vi "Get XY.vi"(8 "error in":errorcluster, 10 "device name":tag) -> (0 "error out":errorcluster, 2 "Y":dbl, 3 "X":dbl)   [LabVIEW 2015]
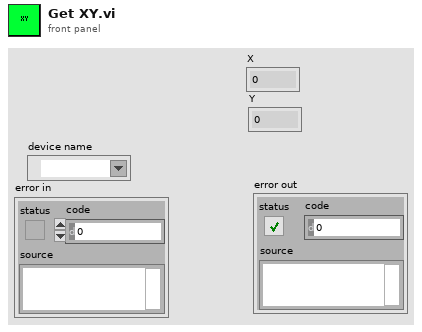
[diagram p1: front panel]
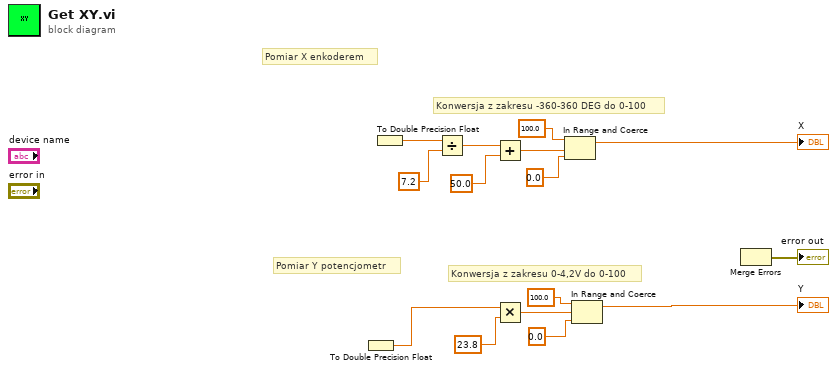
[diagram p0: block diagram]
diagram:
  # "Konwersja z zakresu 0-4,2V do 0-100"
  # "Konwersja z zakresu -360-360 DEG do 0-100"
  # "Pomiar Y potencjometr"
  # "Pomiar X enkoderem"
  n1 = To Double Precision Float() -> (double precision float=w11:dbl)  [unwired: 1 in]
  n2 = To Double Precision Float() -> (double precision float=w15:dbl)  [unwired: 1 in]
  n3 = Divide(x=w15, y=7.2) -> (x/y=w13:dbl)
  n4 = Add(x=w13, y=50.0) -> (x+y=w8:dbl)
  n5 = Multiply(x=w11, y=23.8) -> (x*y=w5:dbl)
  n6 = In Range and Coerce(upper limit=100.0, x=w8, lower limit=0.0) -> (coerced(x)=→"X":dbl)  [unwired: 1 out]
  n7 = In Range and Coerce(upper limit=100.0, x=w5, lower limit=0.0) -> (coerced(x)=→"Y":dbl)  [unwired: 1 out]
  n8 = Merge Errors() -> (→"error out":errorcluster)  [unwired: 2 in]
